vi "get AOI.vi"(8 "error in (no error)":errorcluster, 11 "Thorcam in":refnum<class "Thorcam.lvclass">) -> (0 "error out":errorcluster, 3 "Thorcam out":refnum<class "Thorcam.lvclass">)   [LabVIEW 2012, in "Thorcam.lvclass"]
uses:
  Thorcam.lvclass
  AOI.ctl
  Thorcam.lvclass/Thorcam.ctl
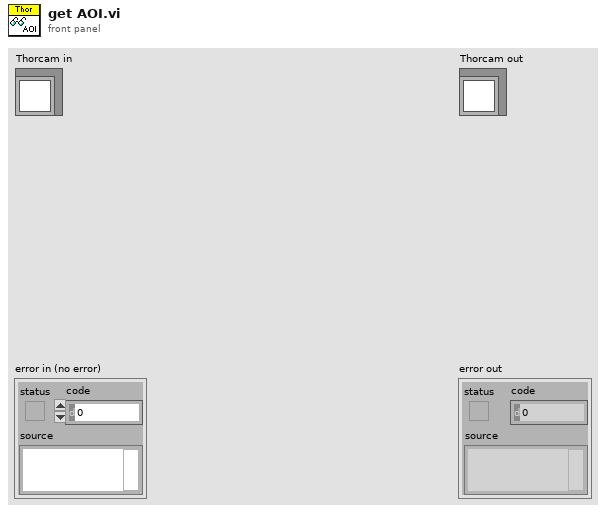
[diagram p1: front panel]
types:
  T1 = typedef "Thorcam.lvclass/AOI.ctl" = cluster{"width":i32, "height":i32, "x pos":i32, "y pos":i32}
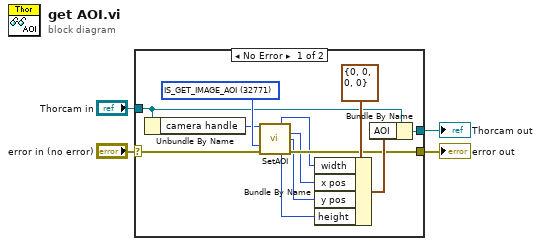
[diagram p0: block diagram]
diagram:
  n1 = case shown="No Error" "error in (no error)" {
    selector: "error in (no error)" -> [w14 w18]
    tunnel: [w11 w18] -> w3
    tunnel: [w9 w17] -> w1
    tunnel: "Thorcam in" -> [w10 w17]
    frame No Error {
      w16 = 32771 items=["IS_SET_IMAGE_AOI"=32770, "IS_GET_IMAGE_AOI"=32771] ("Mode")
      n2 = Unbundle By Name(w10) -> ("camera handle"=w15:u32)
      n3 = call <instrlib>:"SetAOI.vi"("Camera Handle In"=w15, "Mode"=w16, "error in"=w14) -> ("Width Out"=w8:i32, "XPos Out"=w7:i32, "YPos Out"=w6:i32, "Height Out"=w5:i32, "error out"=w11:errorcluster)  [unwired: 7 in, 1 out]
      n4 = Bundle By Name(cluster=T1 {"width"=0, "height"=0, "x pos"=0, "y pos"=0} ("AOI"), "width"=w8, "x pos"=w7, "y pos"=w6, "height"=w5) -> (w13:T1)
      n5 = Bundle By Name(cluster=w10, "AOI"=w13) -> (w9:refnum<class "Thorcam.lvclass">)
    }
    frame Error {
    }
  }
  "error out" <- w3
  "Thorcam out" <- w1
